vi "Emphasize Colo2r.vi"(2 "error in (no error)":errorcluster, 3 "Color":i8, 4 "Image Dst":T1, 5 "Image Src":T1) -> (0 "error out":errorcluster, 1 "Image Out":T1)   [LabVIEW 2009, in "ImageProcessing.lvlib"]
doc: "Output is a grayscaled image calculated as\n (255*X)/(R+G+B) \nwhere X is R, G or B depending on what number is showsen in color (0 = R, 1 = G, 2 = B)."
uses:
  ImageProcessing.lvlib
  <vilib>/vision/Image Controls.llb/IMAQ Image.ctl
  <vilib>/Analysis/Matrix/Numeric/Conversions/Matrix To Array - RM.vi
  <vilib>/Analysis/Matrix/Numeric/Multiply/Multiply - RM,R.vi
  <vilib>/Analysis/Matrix/Numeric/Add/Add - RM,RM.vi
  <vilib>/Analysis/Matrix/Numeric/Conversions/Array To Matrix - RA2.vi
  <vilib>/Analysis/Matrix/NI_Matrix.lvlib
  <vilib>/vision/NI_Vision_Development_Module.lvlib
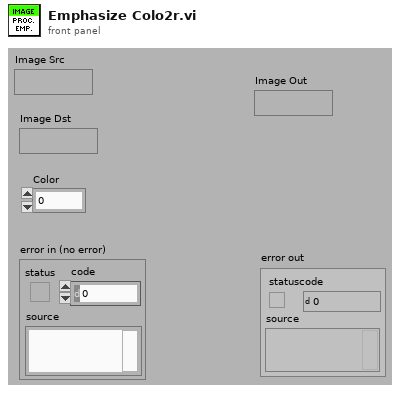
[diagram p1: front panel]
types:
  T1 = typedef "IMAQ Image.ctl" = refnum<image>
  T2 = typedef "NI_Matrix.lvlib/RealMatrix.ctl" = dbl[][]
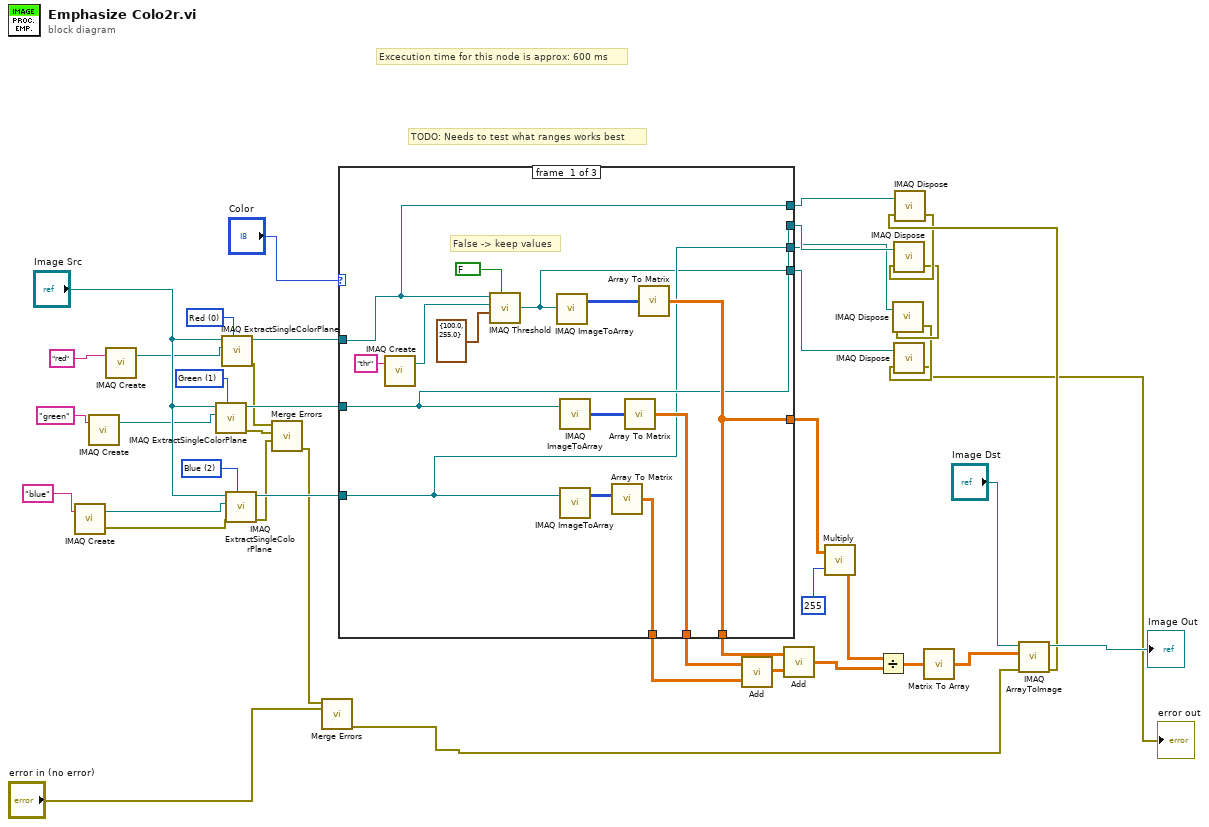
[diagram p0: block diagram]
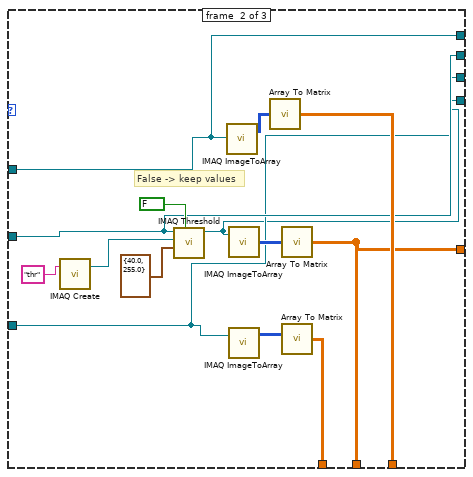
[diagram p2: hidden frame]
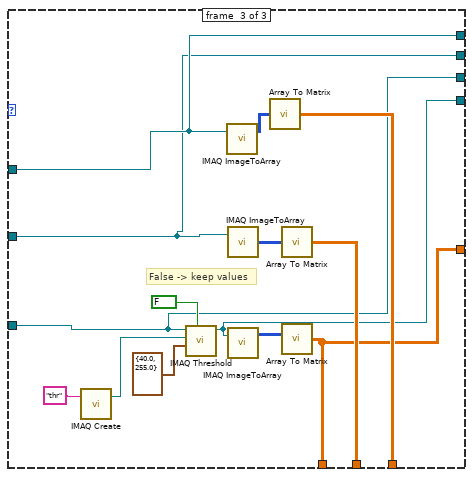
[diagram p3: hidden frame]
diagram:
  w31 = 2 items=["Red", "Green", "Blue", "Hue", "Saturation", "Luminance", "Value", "Intensity"] ("Color Plane")
  w30 = 1 items=["Red", "Green", "Blue", "Hue", "Saturation", "Luminance", "Value", "Intensity"] ("Color Plane")
  w29 = 0 items=["Red", "Green", "Blue", "Hue", "Saturation", "Luminance", "Value", "Intensity"] ("Color Plane")
  # "Excecution time for this node is approx: 600 ms"
  # "TODO: Needs to test what ranges works best"
  n1 = call "IMAQ Create"("Image Name"="blue") -> ("New Image"=w25:T1, "error out"=w19:errorcluster)  [unwired: 3 in, 1 out]
  n2 = call "IMAQ Create"("Image Name"="green") -> ("New Image"=w26:T1)  [unwired: 3 in, 2 out]
  n3 = call "IMAQ Create"("Image Name"="red") -> ("New Image"=w27:T1)  [unwired: 3 in, 2 out]
  n4 = call "IMAQ ExtractSingleColorPlane"("Color Plane"=w30, "Image Dst"=w26, "Image Src"="Image Src") -> ("error out"=w17:errorcluster, "Image Dst Out"=w24:T1)  [unwired: 7 in]
  n5 = call "IMAQ ExtractSingleColorPlane"("Color Plane"=w29, "Image Dst"=w27, "Image Src"="Image Src") -> ("error out"=w16:errorcluster, "Image Dst Out"=w12:T1)  [unwired: 7 in]
  n6 = call "IMAQ ExtractSingleColorPlane"("Color Plane"=w31, "error in (no error)"=w19, "Image Dst"=w25, "Image Src"="Image Src") -> ("error out"=w18:errorcluster, "Image Dst Out"=w23:T1)  [unwired: 6 in]
  n7 = call <vilib>:"Merge Errors.vi"("error in 3 (no error)"=w18, "error in 2 (no error)"=w17, "error in 1 (no error)"=w16) -> ("error out"=w13:errorcluster)  [unwired: 4 in]
  n8 = call <vilib>:"Merge Errors.vi"("error in 2 (no error)"="error in (no error)", "error in 1 (no error)"=w13) -> ("error out"=w14:errorcluster)  [unwired: 5 in]
  n9 = case shown="..0" "Color" {
    tunnel: [w49 w65 w79] -> w32
    tunnel: w12 -> [w46 w60 w74]
    tunnel: w24 -> [w45 w59 w73]
    tunnel: w23 -> [w44 w58 w72]
    tunnel: [w56 w70 w79] -> w20
    tunnel: [w55 w65 w84] -> w21
    tunnel: [w49 w67 w81] -> w22
    tunnel: [w46 w60 w74] -> w9
    tunnel: [w45 w59 w73] -> w8
    tunnel: [w44 w58 w72] -> w7
    tunnel: [w43 w57 w71] -> w6
    frame #0 {
      # "False -> keep values"
      n10 = call "IMAQ Create"("Image Name"="thr") -> ("New Image"=w50:T1)  [unwired: 3 in, 2 out]
      n11 = call "IMAQ Threshold"("Keep/Replace Value (Replace)"=FALSE, "Range"=cluster{"Lower value":sgl, "Upper value":sgl} {"Lower value"=100.0, "Upper value"=255.0}, "Image Dst"=w50, "Image Src"=w46) -> ("Image Dst Out"=w43:T1)  [unwired: 6 in, 1 out]
      n12 = call "IMAQ ImageToArray"("Image"=w43) -> ("Image Pixels (U8)"=w47:u8[][])  [unwired: 3 in, 4 out]
      n13 = call "IMAQ ImageToArray"("Image"=w45) -> ("Image Pixels (U8)"=w53:u8[][])  [unwired: 3 in, 4 out]
      n14 = call "IMAQ ImageToArray"("Image"=w44) -> ("Image Pixels (U8)"=w52:u8[][])  [unwired: 3 in, 4 out]
      n15 = call-poly <vilib>:"Array To Matrix.vi"("Real 2D Array"=w52) -> ("Real Matrix"=w56:T2)
      n16 = call-poly <vilib>:"Array To Matrix.vi"("Real 2D Array"=w53) -> ("Real Matrix"=w55:T2)
      n17 = call-poly <vilib>:"Array To Matrix.vi"("Real 2D Array"=w47) -> ("Real Matrix"=w49:T2)
    }
    frame #1 {
      # "False -> keep values"
      n18 = call "IMAQ Create"("Image Name"="thr") -> ("New Image"=w62:T1)  [unwired: 3 in, 2 out]
      n19 = call "IMAQ Threshold"("Keep/Replace Value (Replace)"=FALSE, "Range"=cluster{"Lower value":sgl, "Upper value":sgl} {"Lower value"=40.0, "Upper value"=255.0}, "Image Dst"=w62, "Image Src"=w59) -> ("Image Dst Out"=w57:T1)  [unwired: 6 in, 1 out]
      n20 = call "IMAQ ImageToArray"("Image"=w60) -> ("Image Pixels (U8)"=w66:u8[][])  [unwired: 3 in, 4 out]
      n21 = call "IMAQ ImageToArray"("Image"=w57) -> ("Image Pixels (U8)"=w69:u8[][])  [unwired: 3 in, 4 out]
      n22 = call "IMAQ ImageToArray"("Image"=w58) -> ("Image Pixels (U8)"=w68:u8[][])  [unwired: 3 in, 4 out]
      n23 = call-poly <vilib>:"Array To Matrix.vi"("Real 2D Array"=w66) -> ("Real Matrix"=w67:T2)
      n24 = call-poly <vilib>:"Array To Matrix.vi"("Real 2D Array"=w69) -> ("Real Matrix"=w65:T2)
      n25 = call-poly <vilib>:"Array To Matrix.vi"("Real 2D Array"=w68) -> ("Real Matrix"=w70:T2)
    }
    frame #2 {
      # "False -> keep values"
      n26 = call "IMAQ Create"("Image Name"="thr") -> ("New Image"=w76:T1)  [unwired: 3 in, 2 out]
      n27 = call "IMAQ Threshold"("Keep/Replace Value (Replace)"=FALSE, "Range"=cluster{"Lower value":sgl, "Upper value":sgl} {"Lower value"=40.0, "Upper value"=255.0}, "Image Dst"=w76, "Image Src"=w72) -> ("Image Dst Out"=w71:T1)  [unwired: 6 in, 1 out]
      n28 = call "IMAQ ImageToArray"("Image"=w74) -> ("Image Pixels (U8)"=w80:u8[][])  [unwired: 3 in, 4 out]
      n29 = call "IMAQ ImageToArray"("Image"=w73) -> ("Image Pixels (U8)"=w83:u8[][])  [unwired: 3 in, 4 out]
      n30 = call "IMAQ ImageToArray"("Image"=w71) -> ("Image Pixels (U8)"=w82:u8[][])  [unwired: 3 in, 4 out]
      n31 = call-poly <vilib>:"Array To Matrix.vi"("Real 2D Array"=w80) -> ("Real Matrix"=w81:T2)
      n32 = call-poly <vilib>:"Array To Matrix.vi"("Real 2D Array"=w83) -> ("Real Matrix"=w84:T2)
      n33 = call-poly <vilib>:"Array To Matrix.vi"("Real 2D Array"=w82) -> ("Real Matrix"=w79:T2)
    }
  }
  n34 = call-poly <vilib>:"Add.vi"("Real Matrix B"=w20, "Real Matrix A"=w21) -> ("A + B"=w39:T2)
  n35 = call-poly <vilib>:"Add.vi"("Real Matrix B"=w39, "Real Matrix A"=w22) -> ("A + B"=w37:T2)
  n36 = call-poly <vilib>:"Multiply.vi"("Real Scalar c"=255, "Real Matrix A"=w32) -> ("A * c"=w36:T2)
  n37 = Divide(x=w36, y=w37) -> (x/y=w10:T2)
  n38 = call-poly <vilib>:"Matrix To Array.vi"("Real Matrix"=w10) -> ("Real 2D Array"=w35:dbl[][])
  n39 = call "IMAQ ArrayToImage"("error in (no error)"=w14, "Image Pixels (U8)"=w35, "Image"="Image Dst") -> ("error out"=w5:errorcluster, "Image Out"=→"Image Out":T1)  [unwired: 7 in]
  n40 = call "IMAQ Dispose"("Image"=w9, "error in (no error)"=w5) -> ("error out"=w4:errorcluster)  [unwired: 4 in]
  n41 = call "IMAQ Dispose"("Image"=w8, "error in (no error)"=w4) -> ("error out"=w3:errorcluster)  [unwired: 4 in]
  n42 = call "IMAQ Dispose"("Image"=w7, "error in (no error)"=w3) -> ("error out"=w2:errorcluster)  [unwired: 4 in]
  n43 = call "IMAQ Dispose"("Image"=w6, "error in (no error)"=w2) -> ("error out"=→"error out":errorcluster)  [unwired: 4 in]
